vi "Get SQL formatted value.vi"(8 "error in (no error)":errorcluster, 11 "Column in":refnum<class "By-Value Column.lvclass">) -> (0 "error out":errorcluster, 2 "Formatted Value":string, 3 "Column out":refnum<class "By-Value Column.lvclass">)   [LabVIEW 2020, in "Basic Columns.lvlib" / "By-Value Column.lvclass"]
uses:
  By-Value Column.lvclass
  Basic Columns/Basic Columns/Column Class/Column Parent.lvclass
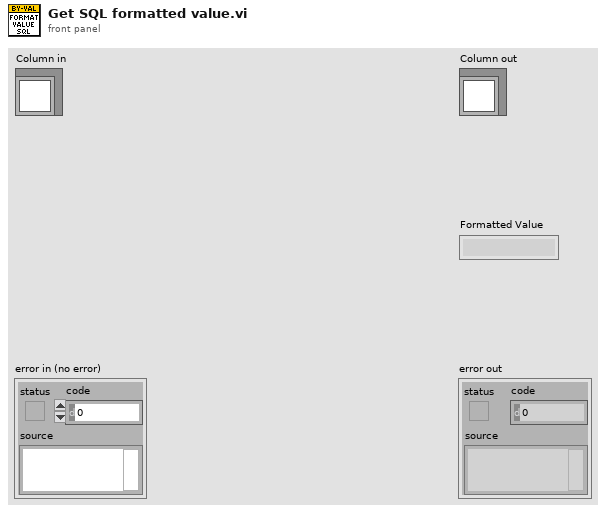
[diagram p1: front panel]
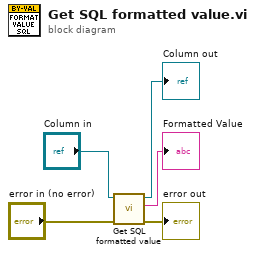
[diagram p0: block diagram]
diagram:
  n1 = call-parent "Get SQL formatted value.vi"("error in (no error)"="error in (no error)", "Column in"="Column in") -> ("error out"=→"error out":errorcluster, "Formatted Value"=→"Formatted Value":string, "Column out"=→"Column out":refnum<class "By-Value Column.lvclass">)  [unwired: 7 in]
